vi "calculaTempoPraBolaEntrarNaArea.vi"(10 "balls":T1[](array[typedef]), 11 "IA State":T2={"our_robots"=[], "enemy_robots"=[], "balls"=[], "geometry"={"field_length"=0, "field_width"=0, "goal_width"=0, "goal_depth"=0, "center_circle_radius"=0, "defense_width"=0, "defense_depth"=0, "free_kick_from_defense_dist"=0, "penalty_spot_from_field_line_dist"=0, "penalty_line_from_spot_dist"=0, "half_moon_depth"=0, "half_moon_width"=0}, "IA Judge"={"stage"="", "command"="", "our_goalie_id"=0.0, "enemy_goalie_id"=0.0, "command enum"=enum."Halt", "Time"=enum."Azul"}, "Received Timestamp"=timestamp(0 s since 1904-01-01), "Events"={"Touch"=FALSE, "id touch"=0.0, "Ball out of \nVision"=FALSE, "Ball inside \nGoalie area"=FALSE, "Robot not responding"=FALSE, "Robots responding status"=[1.0, 1.0, 1.0, 1.0, 1.0, 1.0], "Enemy Ball \nPossession"=FALSE, "Id ini Possession"=0.0, "Ball Possesion"=FALSE, "Id Possesion"=0.0, "Ball at\nour goal side"=FALSE, "Ball at\ntouchline"=FALSE, "Ball at\nenemy goal side"=FALSE}}) -> (3 "Tempo":dbl)   [LabVIEW 2018]
uses:
  Core/AI Input.ctl
  Core/AI Robot.ctl
  Intel/Functions Enum.ctl
  Intel/AttackerStates.ctl
  Path Planning/RRT/PathDests.ctl
  Path Planning/RRT/PathDest.ctl
  Core/AI Ball.ctl
  Core/Field Size.ctl
  Core/AI Judge.ctl
  Intel/Command Enum.ctl
  Util/Events/Events.ctl
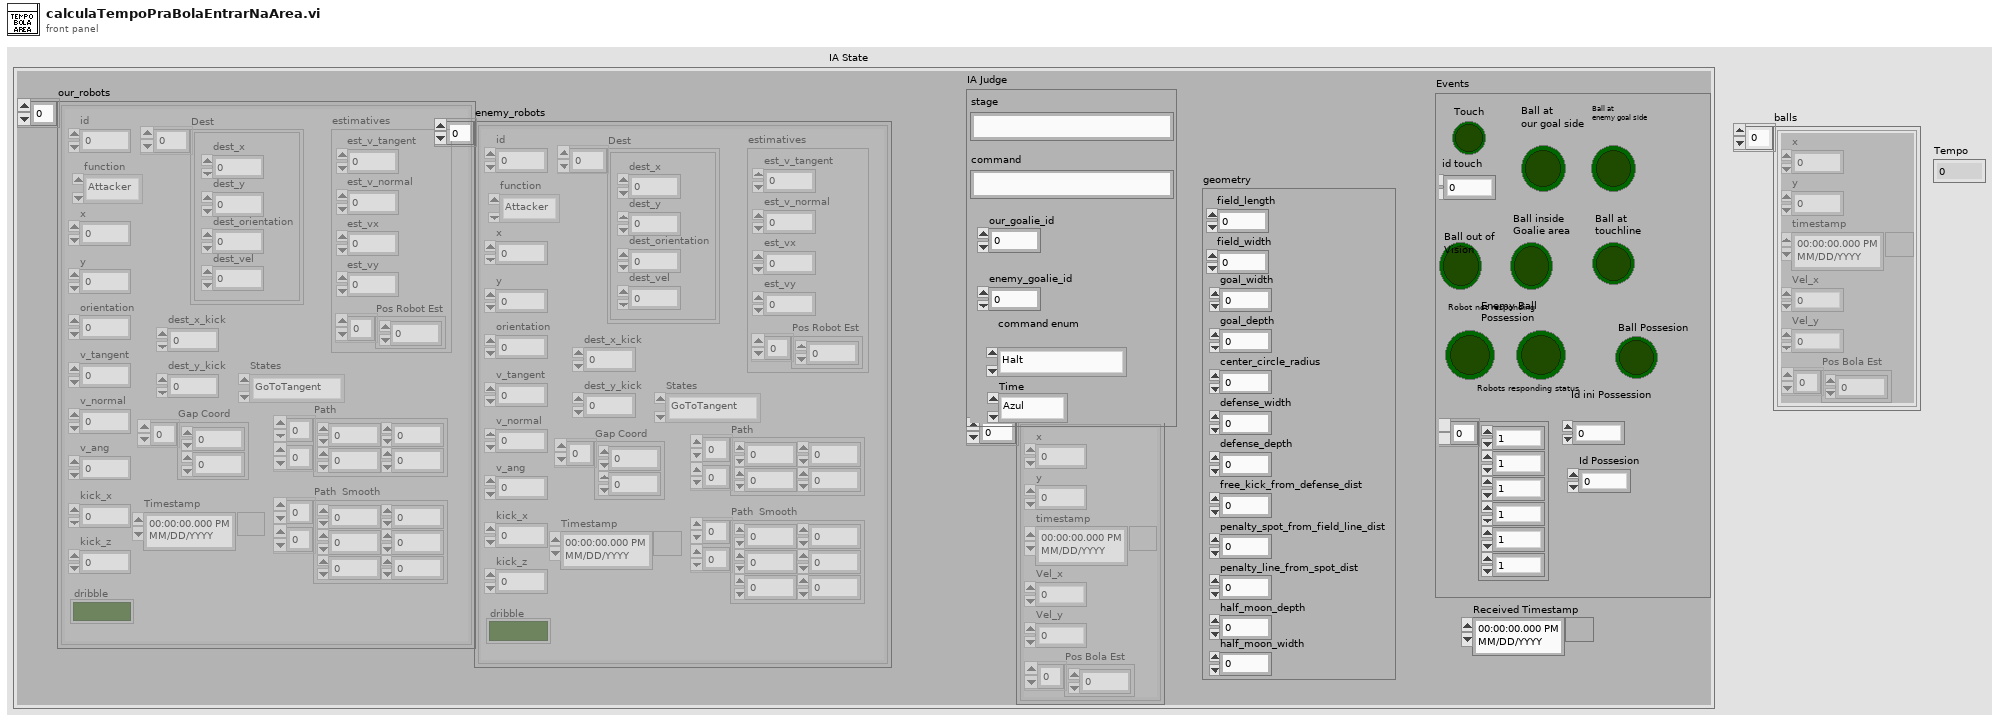
[diagram p1: front panel]
types:
  T1 = typedef "AI Ball.ctl" = cluster{"x":dbl, "y":dbl, "timestamp":timestamp, "Vel_x":dbl, "Vel_y":dbl, "Pos Bola Est":dbl[]}
  T2 = typedef "AI Input.ctl" = cluster{"our_robots":T3[], "enemy_robots":T3[], "balls":T1[], "geometry":T8, "IA Judge":T9, "Received Timestamp":timestamp, "Events":T11}
  T3 = typedef "AI Robot.ctl" = cluster{"id":u32, "function":T4, "x":dbl, "y":dbl, "orientation":dbl, "v_tangent":dbl, "v_normal":dbl, "v_ang":dbl, "kick_x":dbl, "kick_z":dbl, "dribble":bool, "Timestamp":timestamp, "estimatives":cluster{"est_v_tangent":dbl, "est_v_normal":dbl, "est_vx":dbl, "est_vy":dbl, "Pos Robot Est":dbl[]}, "dest_x_kick":dbl, "dest_y_kick":dbl, "Gap Coord":dbl[], "States":T5, "Path ":dbl[][], "Path  Smooth":dbl[][], "Dest":T6}
  T4 = typedef "Functions Enum.ctl" = enum16{"Attacker", "Goalie", "Defender", "Striker", "Goto 0", "Dummy", "Kicker", "ZigZag"}
  T5 = typedef "AttackerStates.ctl" = enum16{"Pass", "GoToTangent", "BallGetting", "GoToKick", "Rotate anti-clockwise", "Rotate Clockwise", ""}
  T6 = typedef "PathDests.ctl" = T7[]
  T7 = typedef "PathDest.ctl" = cluster{"dest_x":dbl, "dest_y":dbl, "dest_orientation":dbl, "dest_vel":dbl}
  T8 = typedef "Field Size.ctl" = cluster{"field_length":u32, "field_width":u32, "goal_width":u32, "goal_depth":u32, "center_circle_radius":u32, "defense_width":u32, "defense_depth":u32, "free_kick_from_defense_dist":u32, "penalty_spot_from_field_line_dist":u32, "penalty_line_from_spot_dist":u32, "half_moon_depth":u32, "half_moon_width":u32}
  T9 = typedef "AI Judge.ctl" = cluster{"stage":string, "command":string, "our_goalie_id":dbl, "enemy_goalie_id":dbl, "command enum":T10, "Time":enum16{"Azul", "Amarelo"}}
  T10 = typedef "Command Enum.ctl" = enum16{"Halt", "Stop", "Force Start", "PKA Normal Start", "Prepare Kickoff Ally", "PKE Normal Start", "Prepare Kickoff Enemy", "Prepare Penalty Ally", "PPA Normal Start", "Prepare Penalty Enemy", "PPE Normal Start", "Ball Placement Enemy Up", "Ball Placement Enemy Down", "Ball Placement Ally Up", "Ball Placement Ally Mid", "Ball Placement Ally Down", "Indirect Free Enemy", "Indirect Free Ally", "Timeout Enemy", "Timeout Ally", "Goal Enemy", "Goal Ally", "Normal Half Time", "Extra Time Break", "Extra Half Time", "None", "Post Game"}
  T11 = typedef "Events.ctl" = cluster{"Touch":bool, "id touch":dbl, "Ball out of \nVision":bool, "Ball inside \nGoalie area":bool, "Robot not responding":bool, "Robots responding status":dbl[], "Enemy Ball \nPossession":bool, "Id ini Possession":dbl, "Ball Possesion":bool, "Id Possesion":dbl, "Ball at\nour goal side":bool, "Ball at\ntouchline":bool, "Ball at\nenemy goal side":bool}
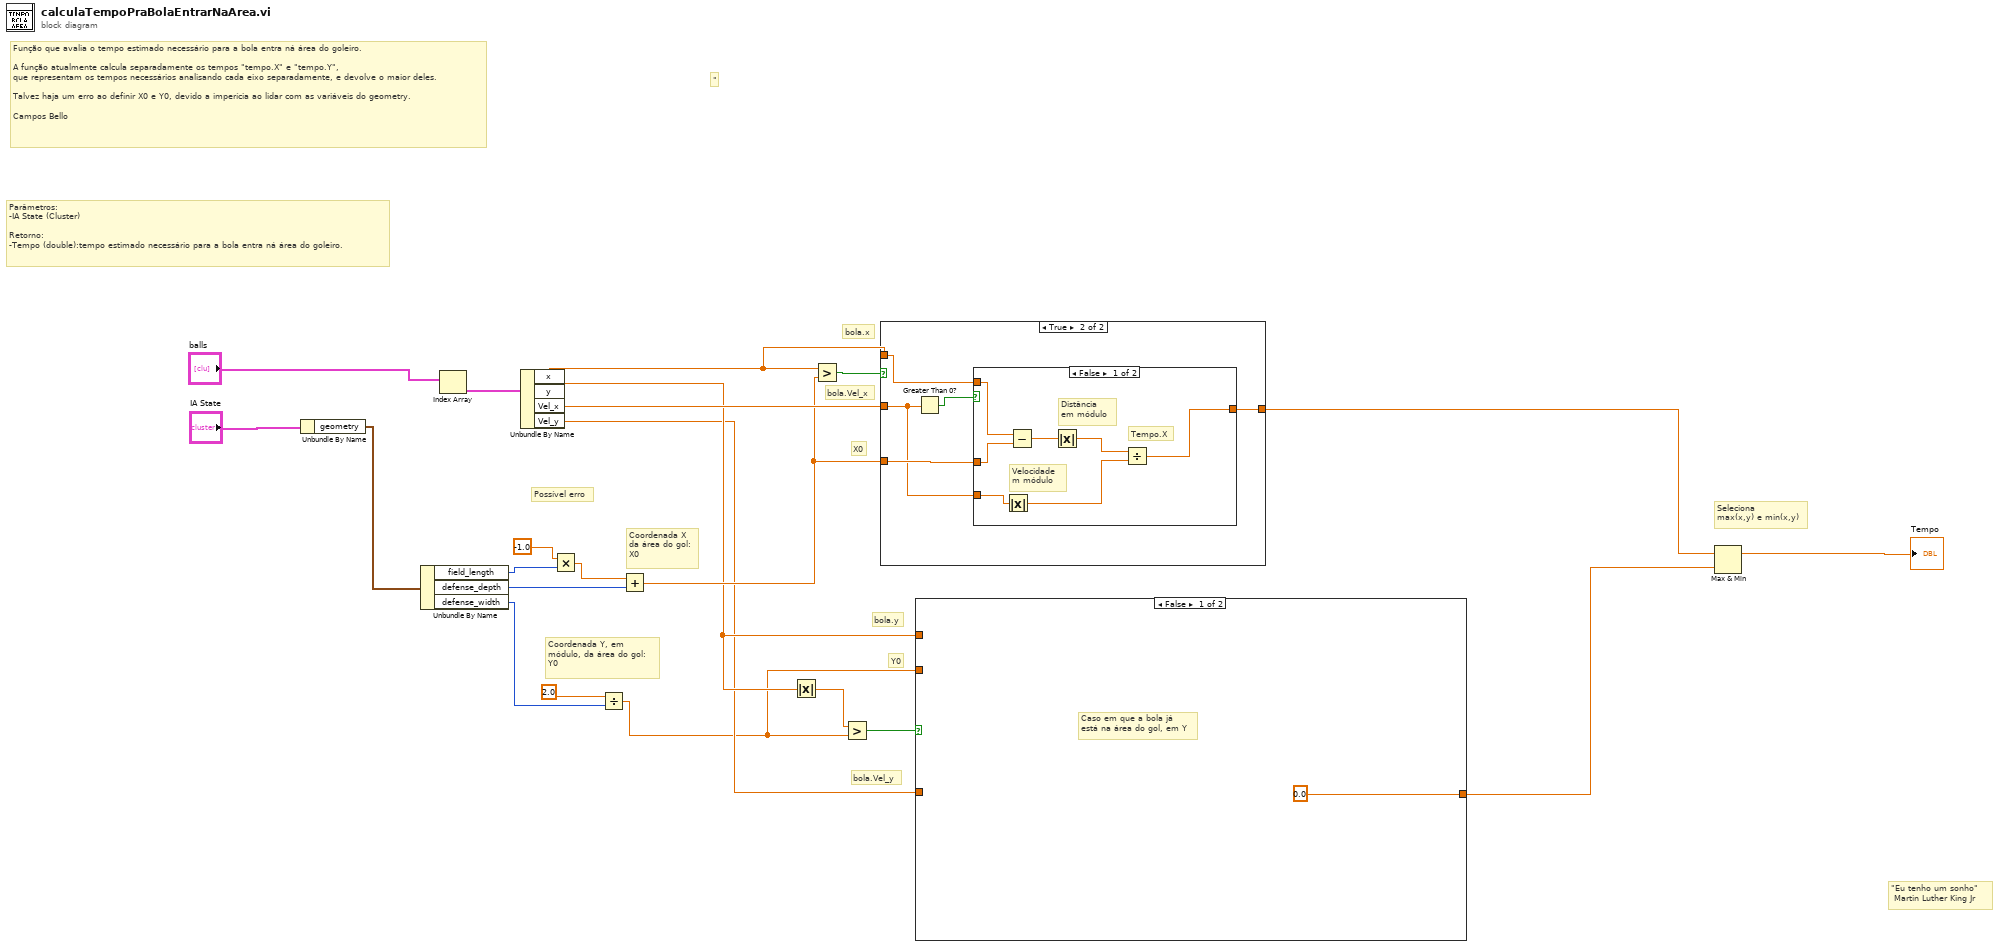
[diagram p0: block diagram]
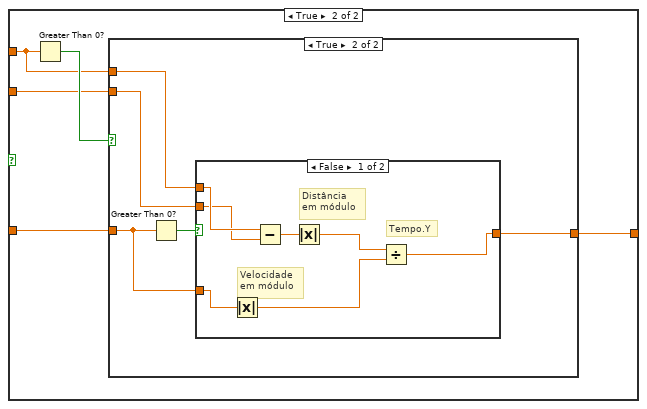
[diagram p2: hidden frame]
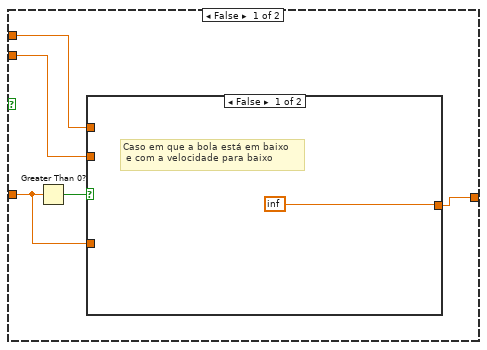
[diagram p3: hidden frame]
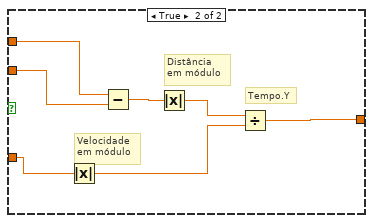
[diagram p4: hidden frame]
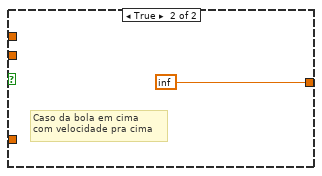
[diagram p5: hidden frame]
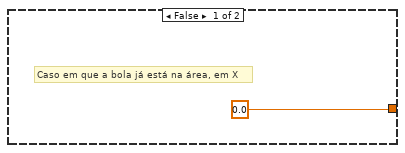
[diagram p6: hidden frame]
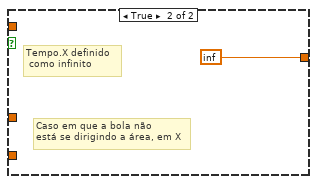
[diagram p7: hidden frame]
diagram:
  # "\"Eu tenho um sonho\"\n Martin Luther King Jr"
  # "\""
  # "Parâmetros:\n-IA State (Cluster)\n\nRetorno:\n-Tempo (double):tempo estimado necessário para a bola entra ná área do goleiro."
  # "Possível erro"
  # "Função que avalia o tempo estimado necessário para a bola entra ná área do goleiro.\n\nA função atualmente calcula separadamente os tempos \"tempo.X\" e \"tempo.Y\", \nque representam os tempos necessários analisando cada eixo separadamente, e devolve o maior deles.\n\nTalvez haja um erro ao definir X0 e Y0, devido a imperícia ao lidar com as variáveis do geometry.\n\nCampos Bello"
  # "X0"
  # "bola.Vel_x"
  # "bola.x"
  # "Seleciona \nmax(x,y) e min(x,y)"
  # "bola.Vel_y"
  # "Y0"
  # "bola.y"
  # "Coordenada Y, em \nmódulo, da área do gol:\nY0"
  # "Coordenada X \nda área do gol:\nX0"
  n1 = Unbundle By Name("IA State") -> ("geometry"=w20:T8)
  n2 = Unbundle By Name(w20) -> ("field_length"=w19:u32, "defense_depth"=w17:u32, "defense_width"=w14:u32)
  n3 = Index Array(array="balls") -> (element=w21:T1)  [unwired: 1 in]
  n4 = Unbundle By Name(w21) -> ("x"=w12:dbl, "y"=w9:dbl, "Vel_x"=w13:dbl, "Vel_y"=w8:dbl)
  n5 = Multiply(x=-1.0, y=w19) -> (x*y=w16:dbl)
  n6 = Divide(x=2.0, y=w14) -> (x/y=w6:dbl)
  n7 = Add(x=w16, y=w17) -> (x+y=w11:dbl)
  n8 = Absolute Value(x=w9) -> (abs(x)=w10:dbl)
  n9 = Greater?(x=w12, y=w11) -> (0:w2:bool)
  n10 = Greater?(x=w10, y=w6) -> (0:w7:bool)
  n11 = case shown="True" w2 {
    tunnel: w13 -> [_ w24]
    tunnel: [0.0 w27] -> w5
    tunnel: w12 -> [_ w26]
    tunnel: w11 -> [_ w25]
    frame False {
      # "Caso em que a bola já está na área, em X"
    }
    frame True {
      n12 = Greater Than 0?(x=w24) -> (x > 0?=w28:bool)
      n13 = case shown="False" w28 {
        tunnel: [w29 inf] -> w27
        tunnel: w26 -> [w35 _]
        tunnel: w25 -> [w34 _]
        tunnel: w24 -> [w33 _]
        frame False {
          # "Velocidade \nm módulo"
          # "Distância \nem módulo"
          # "Tempo.X"
          n14 = Absolute Value(x=w33) -> (abs(x)=w30:dbl)
          n15 = Subtract(x=w35, y=w34) -> (x-y=w32:dbl)
          n16 = Absolute Value(x=w32) -> (abs(x)=w31:dbl)
          n17 = Divide(x=w31, y=w30) -> (x/y=w29:dbl)
        }
        frame True {
          # "Caso em que a bola não \nestá se dirigindo a área, em X"
          # "Tempo.X definido\n como infinito"
        }
      }
    }
  }
  n18 = case shown="False" w7 {
    tunnel: w9 -> [_ w39]
    tunnel: w8 -> [_ w41]
    tunnel: w6 -> [_ w38]
    tunnel: [0.0 w40] -> w4
    frame False {
      # "Caso em que a bola já \nestá na área do gol, em Y"
    }
    frame True {
      n19 = Greater Than 0?(x=w39) -> (x > 0?=w42:bool)
      n20 = case shown="True" w42 {
        tunnel: w41 -> [w44 w56]
        tunnel: [w43 w59] -> w40
        tunnel: w39 -> [w46 w58]
        tunnel: w38 -> [w45 w57]
        frame False {
          n21 = Greater Than 0?(x=w44) -> (x > 0?=w47:bool)
          n22 = case shown="False" w47 {
            tunnel: w46 -> [_ w52]
            tunnel: w45 -> [_ w51]
            tunnel: w44 -> [_ w50]
            tunnel: [inf w49] -> w43
            frame False {
              # "Caso em que a bola está em baixo\n e com a velocidade para baixo"
            }
            frame True {
              # "Velocidade\nem módulo"
              # "Distância \nem módulo"
              # "Tempo.Y"
              n23 = Absolute Value(x=w50) -> (abs(x)=w53:dbl)
              n24 = Subtract(x=w52, y=w51) -> (x-y=w55:dbl)
              n25 = Absolute Value(x=w55) -> (abs(x)=w54:dbl)
              n26 = Divide(x=w54, y=w53) -> (x/y=w49:dbl)
            }
          }
        }
        frame True {
          n27 = Greater Than 0?(x=w56) -> (x > 0?=w60:bool)
          n28 = case shown="False" w60 {
            tunnel: [w61 inf] -> w59
            tunnel: w58 -> [w64 _]
            tunnel: w57 -> [w63 _]
            tunnel: w56 -> [w62 _]
            frame False {
              # "Velocidade\nem módulo"
              # "Distância \nem módulo"
              # "Tempo.Y"
              n29 = Absolute Value(x=w62) -> (abs(x)=w65:dbl)
              n30 = Subtract(x=w64, y=w63) -> (x-y=w67:dbl)
              n31 = Absolute Value(x=w67) -> (abs(x)=w66:dbl)
              n32 = Divide(x=w66, y=w65) -> (x/y=w61:dbl)
            }
            frame True {
              # "Caso da bola em cima \ncom velocidade pra cima"
            }
          }
        }
      }
    }
  }
  n33 = Max & Min(x=w5, y=w4) -> (max(x,y)=→"Tempo":dbl)  [unwired: 1 out]
